vi "write into binary.vi"() -> ()   [LabVIEW 2012]
uses:
  <vilib>/rvi/interface/nirviOpenFPGA/nirviOpenFPGA.xnode
  <vilib>/rvi/interface/nirviMethod/nirviMethod.xnode
  <vilib>/rvi/errors/niLvFpgaMergeErrorWithErrorCode.vi
  <vilib>/ptbypt/NI_PtbyPt.lvlib
  <vilib>/rvi/interface/nirviCloseFPGA/nirviCloseFPGA.xnode
  <vilib>/rvi/interface/nirviReadWriteControl/nirviReadWriteControl.xnode
  <vilib>/rvi/interface/Simulation/niFpgaSimulationCallBeginRW.vi
  <vilib>/rvi/errors/niLvFpgaAdjustHostInterfaceError.vi
  <vilib>/FPGAPlugInAG/Dynamic/niLvFpga_Run_Dynamic.vi
  FPGA Bitfiles/Mockup_FPGATarget_TopLevelFPGAtryw_gkKwyDHwWeY.lvbitx
  <vilib>/FPGAPlugInAG/Dynamic/niLvFpga_StartFifo_Dynamic.vi
  <vilib>/LabVIEW Targets/FPGA/FlexRIO/CustomFPGAMethods/79XXR_Method_IOModuleStatusImpl.vi
  <vilib>/FPGAPlugInAG/Dynamic/niLvFpga_Close_Dynamic.vi
  <vilib>/FPGAPlugInAG/PXI-7951R/niLvFpga_Open_PXI-7951R.vi
  <vilib>/rvi/interface/common/dynamic/niFpgaDynamicAddResources.vi
  <vilib>/FPGAPlugInAG/Dynamic/niLvFpga_ConfigureFifo_Dynamic.vi
  <vilib>/FPGAPlugInAG/Dynamic/niLvFpga_ReadFifo_Dynamic.vi
  <vilib>/userdefined/High Color/nirio_resource_hc.ctl
panel:
  in  "det_type":string[](array[string])
  in  "voltage":string[](array[string])
  in  "Serial numbers":string[](array[string])
  in  "Sources":string[](array[string])
  in  "stop 2":bool
  in  "show_trigger_position_for_debugging":bool
  in  "PXI address":T1 caption="RIO Device"
  in  "Channel 8":bool caption="Channel 1"
  in  "Channel 7":bool caption="Channel 1"
  in  "Channel 6":bool caption="Channel 1"
  in  "Channel 5":bool caption="Channel 1"
  in  "Channel 4":bool caption="Channel 1"
  in  "Channel 3":bool caption="Channel 1"
  in  "Channel 2":bool caption="Channel 1"
  in  "Channel 1":bool
  out "XML String":string
  in  "Trigger":i16[](array[numeric])=[4000, 4000, 4000, 4000, 4000, 4000, 4000, 4000]
  in  "number_of_arrays_per_file":u32=1000
  in  "File Path":path=path "D:/Users/mkurz/Desktop/test data from the FPGA/data from the new program of Drew"
  out "error out":errorcluster
  in  "samples_dataonly":u32=95
  in  "with dead time":bool
  in  "circular buffer length":u32=1000
  in  "pretrigger_samples":u32=15
  in  "number_of_samples_per_array":u32=500000 format="%.2p"
  in  "Simulate":bool
  in  "stop":bool
  out "Elements in FIFO":u32(graph)
  out "Data":i16[](graph)
  out "Inst. Throughput":dbl format="%#_6p"
  out "Loop Time":u32
  in  "read_rate_ms":u32=50
  out "Average Throughput":dbl(graph)
  in  "Write to Disk":bool
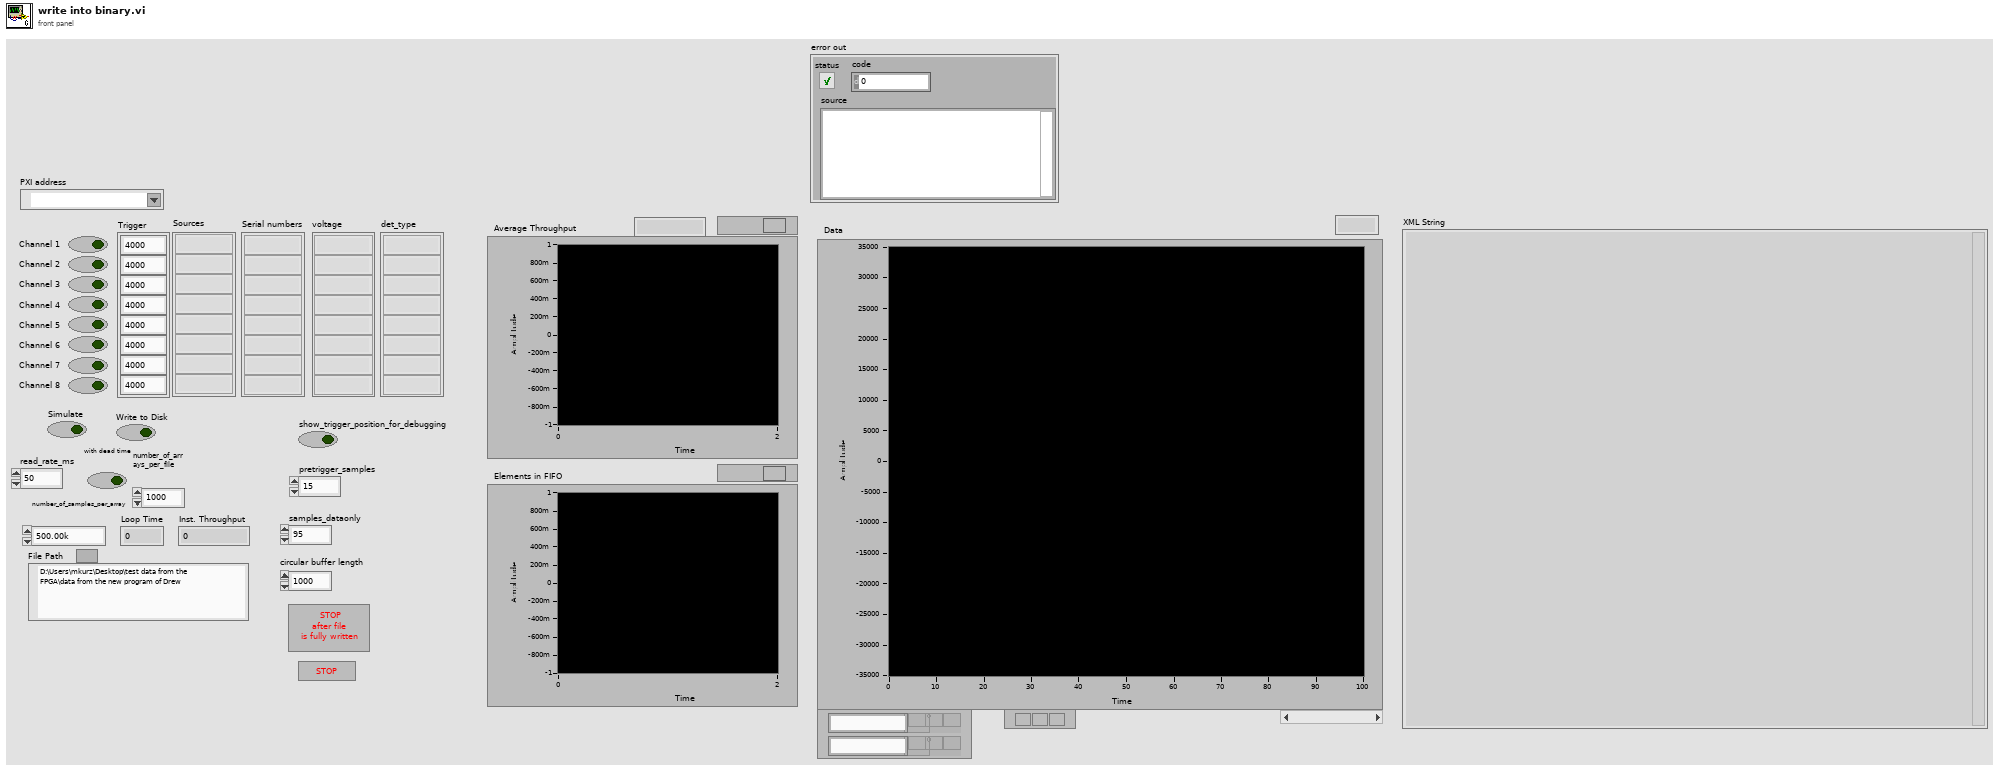
[diagram p1: front panel]
types:
  T1 = typedef "nirio_resource_hc.ctl" = tag
  T2 = enum16{"open", "replace", "create", "open or create", "replace or create", "replace or create with confirmation"}
  T3 = enum16{"big-endian, network order", "native, host order", "little-endian"}
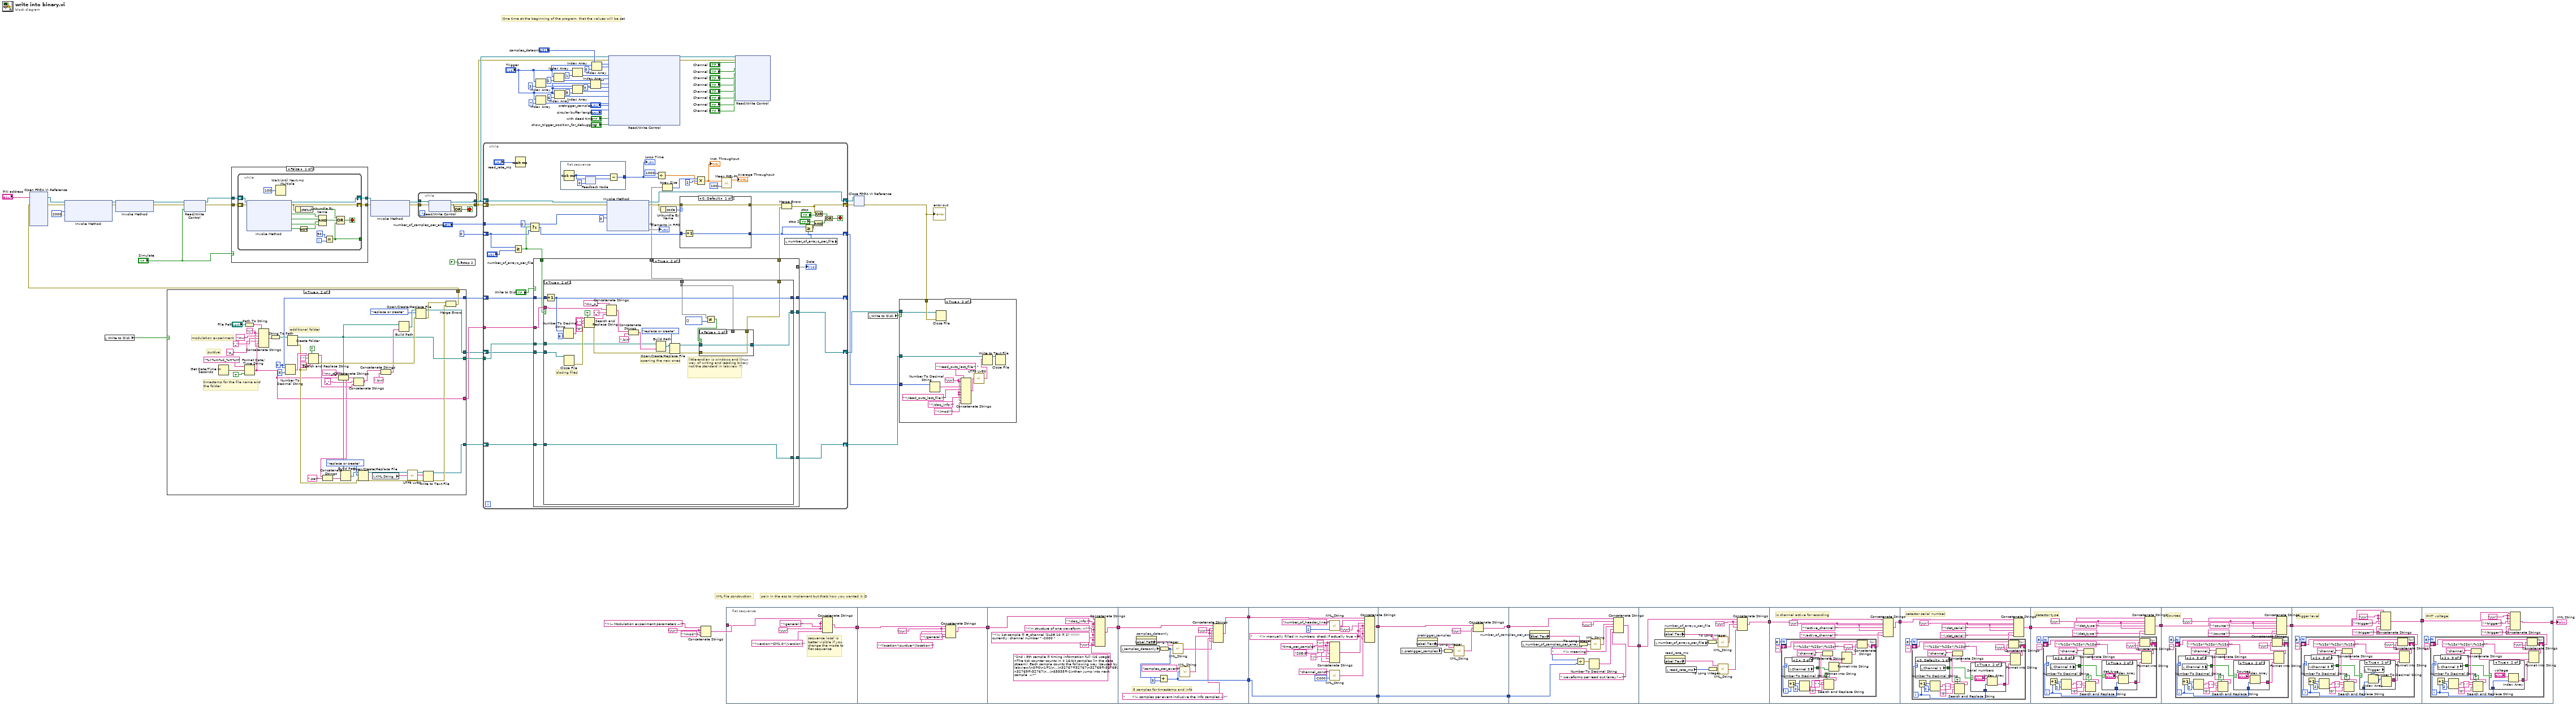
[diagram p0: block diagram]
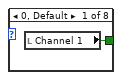
[diagram p2: hidden frame]
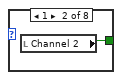
[diagram p3: hidden frame]
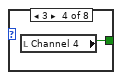
[diagram p4: hidden frame]
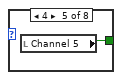
[diagram p5: hidden frame]
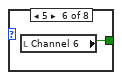
[diagram p6: hidden frame]
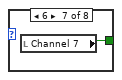
[diagram p7: hidden frame]
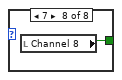
[diagram p8: hidden frame]
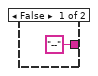
[diagram p9: hidden frame]
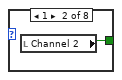
[diagram p10: hidden frame]
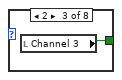
[diagram p11: hidden frame]
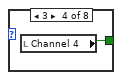
[diagram p12: hidden frame]
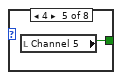
[diagram p13: hidden frame]
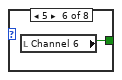
[diagram p14: hidden frame]
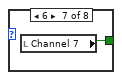
[diagram p15: hidden frame]
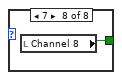
[diagram p16: hidden frame]
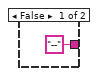
[diagram p17: hidden frame]
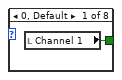
[diagram p18: hidden frame]
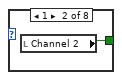
[diagram p19: hidden frame]
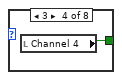
[diagram p20: hidden frame]
diagram:
  w22 = "\r\n"
  # "pain in the ass to implement but thats how you wanted it :D"
  # "XML file construction"
  # "One time at the beginning of the program, that the values will be set"
  n1 = local read "Write to Disk"() -> (w65:bool)
  n2 = case shown="True" w65 {
    tunnel: [_ w107] -> w70
    tunnel: [_ w95] -> w69
    tunnel: [_ w109] -> w68
    tunnel: [_ w115] -> w66
    tunnel: [_ w111] -> w64
    tunnel: [_ w97] -> w62
    frame False {
    }
    frame True {
      w115 = 0 ("number")
      w96 = "\\" ("string")
      # "modulation experiment"
      # "purdue"
      # "timestamp for the file name and the folder"
      # "additional folder"
      n3 = Get Date/Time In Seconds() -> (seconds since 1Jan1904=w124:timestamp)
      n4 = Path To String(path="File Path") -> (string=w126:string)
      n5 = Format Date/Time String(time format string (%c)="%Y%m%d_%H%M", seconds (now)=w124, UTC format=TRUE) -> (date/time string=w95:string)
      n6 = Concatenate Strings(w126, w96, "mx" ("string"), "_" ("string"), "p_" ("string"), w95, w96) -> (w129:string)
      n7 = String To Path(string=w129) -> (path=w130:path)
      n8 = Number To Decimal String(number=w115, width (-)=i16 6) -> (decimal integer string=w119:string)
      n9 = Create Folder(path (use dialog)=w130) -> (created path=w107:path, error out=w105:errorcluster)  [unwired: 2 in, 1 out]
      n10 = Search and Replace String(replace all?=TRUE ("replace all? (F)"), input string=w119, search string=" ", replace string="0" ("replace string (\"\")"), error in=w105) -> (result string=w91:string, error out=w113:errorcluster)  [unwired: 3 in, 2 out]
      n11 = Concatenate Strings("mx_p_" ("string"), w95) -> (w92:string)
      n12 = Concatenate Strings(w92, ".par" ("substring (\"\")")) -> (w102:string)
      n13 = Build Path(base path=w107, name or relative path=w102) -> (appended path=w108:path)
      n14 = Concatenate Strings(w92, "_" ("string"), w91) -> (w93:string)
      n15 = Open/Create/Replace File(file path (use dialog)=w108, error in=w105, operation (0:open)=T2."replace or create") -> (refnum out=w98:refnum<file>, error out=w100:errorcluster)  [unwired: 3 in, 1 out]
      n16 = local read "XML String"() -> (w88:string)
      n17 = Concatenate Strings(w93, ".bin" ("substring (\"\")")) -> (w104:string)
      n18 = Build Path(base path=w107, name or relative path=w104) -> (appended path=w114:path)
      n19 = call "UTF8 LV80.vi"("text"=w88) -> ("utf-8 text out"=w89:string)
      n20 = Open/Create/Replace File(file path (use dialog)=w114, error in=w113, operation (0:open)=T2."replace or create") -> (refnum out=w111:refnum<file>, error out=w110:errorcluster)  [unwired: 3 in, 1 out]
      n21 = Write to Text File(file (use dialog)=w98, text=w89, error in=w100) -> (refnum out=w97:refnum<file>, error out=w99:errorcluster)  [unwired: 1 in, 1 out]
      n22 = Merge Errors(w110, w99) -> (w109:errorcluster)
    }
  }
  n23 = xnode "Open FPGA VI Reference"("error in"=w68, "resource name"="PXI address") -> ("FPGA VI Reference Out"=w83:refnum<k20>, "error out"=w82:errorcluster)
  n24 = xnode "Invoke Method"("FPGA VI Reference In"=w83, "error in"=w82, "Requested Depth"=u32 20000000) -> ("FPGA VI Reference Out"=w85:refnum<k20>, "error out"=w84:errorcluster)  [unwired: 1 out]
  n25 = xnode "Invoke Method"("FPGA VI Reference In"=w85, "error in"=w84) -> ("FPGA VI Reference Out"=w77:refnum<k20>, "error out"=w76:errorcluster)
  n26 = xnode "Read/Write Control"("FPGA VI Reference In"=w77, "error in"=w76, "Simulate"="Simulate") -> ("FPGA VI Reference Out"=w42:refnum<k20>, "error out"=w41:errorcluster)
  n27 = case shown="False" "Simulate" {
    tunnel: [w134 w152] -> w78
    tunnel: [w133 w151] -> w79
    tunnel: w42 -> [w132 w152]
    tunnel: w41 -> [w131 w151]
    frame False {
      n28 = while {
        shift-right: [w141] -> w133
        shift-left: w131 -> [w149]
        shift-right: [w148] -> w134
        shift-left: w132 -> [w150]
        tunnel: [w137] -> _
        i -> [w143]
        stop <- w138 stop-if-true
        n29 = xnode "Invoke Method"("FPGA VI Reference In"=w150, "error in"=w149) -> ("FPGA VI Reference Out"=w148:refnum<k20>, "error out"=w141:errorcluster, "IO Module Present?"=w147:bool, "Power Enabled?"=w146:bool, "IO Enabled?"=w145:bool, "IO Module Mismatch?"=w136:bool)
        n30 = Wait Until Next ms Multiple(millisecond multiple=u32 100) -> ()  [unwired: 1 out]
        n31 = Unbundle By Name(w141) -> ("status"=w140:bool)
        n32 = Not(x=w136) -> (.not. x?=w135:bool)
        n33 = Compound Arithmetic op=AND(w147, w146, w145, w135) -> (w139:bool)
        n34 = Equal?(x=50, y=w143) -> (x = y?=w137:bool)
        n35 = Compound Arithmetic op=OR(w140, w139, w137) -> (w138:bool)
      }
    }
    frame True {
    }
  }
  n36 = xnode "Invoke Method"("FPGA VI Reference In"=w78, "error in"=w79) -> ("FPGA VI Reference Out"=w80:refnum<k20>, "error out"=w81:errorcluster)  [unwired: 1 in]
  n37 = while {
    tunnel: [w153] -> w25
    tunnel: [w158] -> w26
    tunnel: w80 -> [w157]
    tunnel: w81 -> [w156]
    stop <- w154 stop-if-true
    n38 = xnode "Read/Write Control"("FPGA VI Reference In"=w157, "error in"=w156) -> ("FPGA VI Reference Out"=w158:refnum<k20>, "error out"=w153:errorcluster, "Init Done"=w155)
    n39 = Or(x=w153, y=w155) -> (x .or. y?=w154:bool)
  }
  n40 = local write "stop 2"(FALSE ("stop 2")) -> ()
  n41 = while {
    shift-right: [w202] -> w87
    shift-left: w26 -> [w186]
    shift-right: [w175] -> w86
    shift-left: w25 -> [w185]
    tunnel: "number_of_samples_per_array" -> [w187]
    tunnel: w69 -> [w183]
    shift-right: [w162] -> w27
    shift-left: u32 0 -> [w182]
    tunnel: w70 -> [w184]
    shift-right: [w177] -> _
    shift-left: w66 -> [w178]
    shift-right: [w172] -> w63
    shift-left: w64 -> [w173]
    shift-right: [w169] -> w61
    shift-left: w62 -> [w170]
    stop <- w159 stop-if-true
    n42 = Greater Or Equal?(x=w182, y="number_of_arrays_per_file") -> (x >= y?=w179:bool)
    n43 = Wait (ms)(milliseconds to wait="read_rate_ms") -> ()  [unwired: 1 out]
    n44 = Select(t=u32 0, s=w179, f=w182) -> (s? t:f=w180:u32)
    n45 = flat-sequence {
      tunnel: [w206] -> w191
      frame #0 {
        n46 = Tick Count (ms)() -> (millisecond timer value=w205:u32)
        n47 = feedback #1(u32 0 ("millisecond timer value")) -> (w204:u32)
        n48 = feedback-in #1(w205) -> ()
        n49 = Subtract(x=w205, y=w204) -> (x-y=w206:u32)
      }
    }
    n50 = xnode "Invoke Method"("FPGA VI Reference In"=w186, "error in"=w185, "Number of Elements"=w187, "Timeout (ms)"=0) -> ("FPGA VI Reference Out"=w202:refnum<k20>, "error out"=w198:errorcluster, "Data"=w166:void[], "Elements Remaining"=→"Elements in FIFO")
    n51 = case shown="True" "Write to Disk" {
      tunnel: w166 -> [w208 w213]
      tunnel: [w208 _] -> w167
      tunnel: w184 -> [_ w221]
      tunnel: w183 -> [_ w220]
      tunnel: w179 -> [_ w219]
      tunnel: w178 -> [w210 w218]
      tunnel: [w210 w217] -> w177
      tunnel: [_ w216] -> w174
      tunnel: [w209 w215] -> w172
      tunnel: w173 -> [w209 w214]
      tunnel: w170 -> [w207 w212]
      tunnel: [w207 w211] -> w169
      frame False {
      }
      frame True {
        n52 = case shown="True" w219 {
          tunnel: w221 -> [_ w241]
          tunnel: w220 -> [_ w246]
          tunnel: w213 -> [w224 w238]
          tunnel: [w222 w236] -> w216
          tunnel: w214 -> [w228 w254]
          tunnel: w218 -> [w229 w256]
          tunnel: [w229 w255] -> w217
          tunnel: [w227 w247] -> w215
          tunnel: w212 -> [w226 w237]
          tunnel: [w226 w237] -> w211
          frame False {
            # "binary writing will write 0 if there is no data"
            n53 = Not Equal?(x=w224, y=i16[] []) -> (x != y?=w223:bool)
            n54 = case shown="False" w223 {
              tunnel: w228 -> [w230 w235]
              tunnel: [w230 w234] -> w227
              tunnel: [_ w233] -> w222
              tunnel: w224 -> [_ w231]
              frame False {
              }
              frame True {
                n55 = Write to Binary File(file (use dialog)=w235, data=w231, 9:T3."little-endian" ("byte order (0:big-endian, network order)")) -> (refnum out=w234:refnum<file>, error out=w233:errorcluster)  [unwired: 3 in, 1 out]
              }
            }
          }
          frame True {
            # "opening the new ones"
            # "closing files"
            # "little-endian is windows and linux way of writing and reading binary not the standard in labview !?!"
            n56 = Increment(x=w256) -> (x+1=w255:i32)
            n57 = Number To Decimal String(number=w255, width (-)=i16 6) -> (decimal integer string=w258:string)
            n58 = Close File(refnum=w254) -> (error out=w253:errorcluster)  [unwired: 1 in, 1 out]
            n59 = Search and Replace String(replace all?=TRUE ("replace all? (F)"), input string=w258, search string=" ", replace string="0" ("replace string (\"\")"), error in=w253) -> (result string=w245:string, error out=w252:errorcluster)  [unwired: 3 in, 2 out]
            n60 = Concatenate Strings("mx_p_" ("string"), w246, "_" ("string"), w245) -> (w242:string)
            n61 = Concatenate Strings(w242, ".bin" ("substring (\"\")")) -> (w243:string)
            n62 = Build Path(base path=w241, name or relative path=w243) -> (appended path=w251:path)
            n63 = Open/Create/Replace File(file path (use dialog)=w251, error in=w252, operation (0:open)=T2."replace or create") -> (refnum out=w248:refnum<file>, error out=w249:errorcluster)  [unwired: 3 in, 1 out]
            n64 = Not Equal?(x=w238, y=i16[] []) -> (x != y?=w239:bool)
            n65 = case shown="False" w239 {
              tunnel: w249 -> [w264 w271]
              tunnel: w248 -> [w265 w270]
              tunnel: [w265 w269] -> w247
              tunnel: [w264 w268] -> w236
              tunnel: w238 -> [_ w267]
              frame False {
              }
              frame True {
                n66 = Write to Binary File(file (use dialog)=w270, data=w267, error in=w271, 9:T3."little-endian" ("byte order (0:big-endian, network order)")) -> (refnum out=w269:refnum<file>, error out=w268:errorcluster)  [unwired: 2 in, 1 out]
              }
            }
          }
        }
      }
    }
    "Data" <- w167
    n67 = Divide(x=u32 1000, y=w191) -> (x/y=w193:dbl)
    n68 = Unbundle By Name(w198) -> ("code"=w199:i32)
    n69 = Array Size(array=w166) -> (size(s)=w197:i32)
    n70 = case shown="0, Default" w199 {
      tunnel: [w274 errorcluster {"status"=FALSE, "code"=0, "source"=""} ("error constant")] -> w176
      tunnel: w198 -> [w274 _]
      tunnel: w180 -> [w273 w275]
      tunnel: [w272 w275] -> w162
      frame 0, Default {
        n71 = Increment(x=w273) -> (x+1=w272:u32)
      }
      frame -50400 {
      }
    }
    n72 = Compound Arithmetic op=MULTIPLY(w197, 2 ("y"), w193) -> (w189:dbl)
    "Inst. Throughput" <- w189
    n73 = call <vilib>:"Mean PtByPt.vi"("x"=w189, "sample length"=100) -> ("mean"=→"Average Throughput":dbl)  [unwired: 2 in, 1 out]
    n74 = Merge Errors(w176, w174) -> (w175:errorcluster)
    n75 = local read "number_of_arrays_per_file"() -> (w165:u32)
    n76 = Greater Or Equal?(x=w162, y=w165) -> (x >= y?=w164:bool)
    n77 = And(x="stop 2", y=w164) -> (x .and. y?=w163:bool)
    n78 = Or(x=w175, y="stop") -> (x .or. y?=w160:bool)
    n79 = Or(x=w160, y=w163) -> (x .or. y?=w159:bool)
    "Loop Time" <- w191
  }
  n80 = Index Array(array="Trigger", index=3) -> (element=w51:i16)
  n81 = Index Array(array="Trigger", index=7) -> (element=w43:i16)
  n82 = Index Array(array="Trigger", index=2) -> (element=w54:i16)
  n83 = Index Array(array="Trigger", index=6) -> (element=w44:i16)
  n84 = Index Array(array="Trigger", index=1) -> (element=w53:i16)
  n85 = Index Array(array="Trigger", index=5) -> (element=w45:i16)
  n86 = Index Array(array="Trigger", index=4) -> (element=w46:i16)
  n87 = Index Array(array="Trigger", index=0) -> (element=w38:i16)
  n88 = xnode "Read/Write Control"("FPGA VI Reference In"=w26, "error in"=w25, "Record Size only data"="samples_dataonly", "Trigger 1"=w38, "Trigger 2"=w53, "Trigger 3"=w54, "Trigger 4"=w51, "Trigger 5"=w46, "Trigger 6"=w45, "Trigger 7"=w44, "Trigger 8"=w43, "# of pretrigger"="pretrigger_samples", "circular buffer length"="circular buffer length", "with dead time"="with dead time", "show_trigger_position_for_debugging"="show_trigger_position_for_debugging") -> ("FPGA VI Reference Out"=w40:refnum<k20>, "error out"=w39:errorcluster)
  n89 = Concatenate Strings("<!-- Modulation experiment parameters -->", w22, w22, "<mod>" ("string")) -> (w23:string)
  n90 = flat-sequence {
    tunnel: w23 -> [w278]
    tunnel: [w280] -> w17
    tunnel: w17 -> [w284]
    tunnel: [w286] -> w16
    tunnel: w16 -> [w287]
    tunnel: [w293] -> w15
    tunnel: w15 -> [w301]
    tunnel: [w302] -> w4
    tunnel: [w297] -> w2
    tunnel: w4 -> [w320]
    tunnel: [w321] -> w3
    tunnel: w2 -> [w322]
    tunnel: [w322] -> w1
    tunnel: w3 -> [w328]
    tunnel: [w327] -> w14
    tunnel: [w323] -> w5
    tunnel: w1 -> [w323]
    tunnel: w14 -> [w338]
    tunnel: [w337] -> w13
    tunnel: w5 -> [w331]
    tunnel: w13 -> [w349]
    tunnel: [w351] -> w12
    tunnel: w12 -> [w361]
    tunnel: [w354] -> w11
    tunnel: w11 -> [w394]
    tunnel: [w387] -> w9
    tunnel: w9 -> [w425]
    tunnel: [w424] -> w8
    tunnel: w8 -> [w462]
    tunnel: [w461] -> w7
    tunnel: [w505] -> w10
    tunnel: w7 -> [w498]
    tunnel: w10 -> [w537]
    tunnel: [w536] -> w6
    frame #0 {
      w277 = "\r\n"
      # "sequence local is better visible if you change the mode to flat sequence"
      n91 = Concatenate Strings(w278, w277, w277, "<general>" ("string"), w277, "<version>CM1.0</version>" ("string")) -> (w280:string)
    }
    frame #1 {
      w283 = "\r\n"
      n92 = Concatenate Strings(w284, w283, "<location>purdue</location>" ("string"), w283, "</general>" ("string")) -> (w286:string)
    }
    frame #2 {
      w288 = "\r\n"
      n93 = Concatenate Strings(w287, w288, w288, "<daq_info>" ("string"), w288, "<!-- structure of one waveform: -->", w288, "<!-- 1st sample = #_channel (2LSB 10 = 2) !!!!!!!! currently: channel number * -2000 " ("string"), w288, "2nd - 5th sample = timing information full I16 usage\nThe tick counter counts in 4 16-bit samples (in the data stream). Each sample counts the following way (caused by labview)\n0=0\n1=1\n…\n32767=32767\n32768=-32768\n32769=-32767\n…\n65535=-1\nthen jump into next sample  -->" ("string"), w288) -> (w293:string)
    }
    frame #3 {
      w294 = "\r\n"
      # "5 samples for timestamp and info"
      n94 = local read "samples_dataonly"() -> (w305:u32)
      n95 = property on="samples_dataonly" class="DigNum (strict)"() -> ("Label.Text"=w304:string)  [unwired: 2 in, 2 out]
      n96 = To Long Integer(number=w305) -> (32bit integer=w299:i32)
      n97 = Add(x=w299, y=5) -> (x+y=w297:i32)
      n98 = call "XML_String.vi"("variable"=w299, "variable name"=w304) -> ("xml string"=w303:string)  [unwired: 1 in]
      n99 = call "XML_String.vi"("variable"=w297, "variable name"="samples_per_event") -> ("xml string"=w296:string)  [unwired: 1 in]
      n100 = Concatenate Strings(w301, w294, w303, w294, w296, "      <!-- samples per event inclusive the info samples -->" ("string"), w294) -> (w302:string)
    }
    frame #4 {
      w313 = ">" ("string")
      w316 = "<" ("string")
      w314 = "time_per_sample" ("variable name")
      w307 = "      <!-- manually filled in numbers, check if actually true -->" ("string")
      w306 = "\r\n"
      n101 = call "XML_String.vi"("variable"=-2000, "variable name"="channel_const") -> ("xml string"=w308:string)  [unwired: 1 in]
      n102 = call "XML_String.vi"("variable"=2, "variable name"="number_of_header_lines") -> ("xml string"=w319:string)  [unwired: 1 in]
      n103 = Concatenate Strings(w316, w314, w313, "20E-9" ("string"), w316, "/" ("string"), w314, w313) -> (w311:string)
      n104 = Concatenate Strings(w320, w319, w307, w306, w311, w307, w306, w308, w307, w306) -> (w321:string)
    }
    frame #5 {
      n105 = local read "pretrigger_samples"() -> (w330:u32)
      n106 = property on="pretrigger_samples" class="DigNum (strict)"() -> ("Label.Text"=w329:string)  [unwired: 2 in, 2 out]
      n107 = To Long Integer(number=w330) -> (32bit integer=w326:i32)
      n108 = call "XML_String.vi"("variable"=w326, "variable name"=w329) -> ("xml string"=w324:string)  [unwired: 1 in]
      n109 = Concatenate Strings(w328, w324, "\r\n") -> (w327:string)
    }
    frame #6 {
      n110 = local read "number_of_samples_per_array"() -> (w335:u32)
      n111 = property on="number_of_samples_per_array" class="DigNum (strict)"() -> ("Label.Text"=w342:string)  [unwired: 2 in, 2 out]
      n112 = Divide(x=w335, y=w331) -> (x/y=w336:dbl)
      n113 = To Long Integer(number=w335) -> (32bit integer=w339:i32)
      n114 = Number To Decimal String(number=w336) -> (decimal integer string=w333:string)  [unwired: 1 in]
      n115 = call "XML_String.vi"("variable"=w339, "variable name"=w342) -> ("xml string"=w341:string)  [unwired: 1 in]
      n116 = Concatenate Strings(w338, "\r\n", w341, "        <!-- meaning " ("string"), w333, " waveforms per read out (array) -->" ("string")) -> (w337:string)
    }
    frame #7 {
      w347 = "\r\n"
      n117 = local read "number_of_arrays_per_file"() -> (w348:u32)
      n118 = property on="number_of_arrays_per_file" class="DigNum (strict)"() -> ("Label.Text"=w353:string)  [unwired: 2 in, 2 out]
      n119 = property on="read_rate_ms" class="DigNum (strict)"() -> ("Label.Text"=w346:string)  [unwired: 2 in, 2 out]
      n120 = local read "read_rate_ms"() -> (w345:u32)
      n121 = To Long Integer(number=w348) -> (32bit integer=w350:i32)
      n122 = To Long Integer(number=w345) -> (32bit integer=w344:i32)
      n123 = call "XML_String.vi"("variable"=w350, "variable name"=w353) -> ("xml string"=w352:string)  [unwired: 1 in]
      n124 = call "XML_String.vi"("variable"=w344, "variable name"=w346) -> ("xml string"=w343:string)  [unwired: 1 in]
      n125 = Concatenate Strings(w349, w347, w352, w347, w343) -> (w351:string)
    }
    frame #8 {
      w358 = "\r\n"
      # "is channel active for recording"
      n126 = for {
        N: 8 -> [_]
        shift-right: [w367] -> w355
        shift-left: "" -> [w368]
        i -> [w366]
        n127 = case shown="2" w366 {
          tunnel: [w379 w380 w381 w382 w383 w384 w385 w386] -> w363
          frame 0, Default {
            n128 = local read "Channel 1"() -> (w379:bool)
          }
          frame 1 {
            n129 = local read "Channel 2"() -> (w380:bool)
          }
          frame 2 {
            n130 = local read "Channel 3"() -> (w381:bool)
          }
          frame 3 {
            n131 = local read "Channel 4"() -> (w382:bool)
          }
          frame 4 {
            n132 = local read "Channel 5"() -> (w383:bool)
          }
          frame 5 {
            n133 = local read "Channel 6"() -> (w384:bool)
          }
          frame 6 {
            n134 = local read "Channel 7"() -> (w385:bool)
          }
          frame 7 {
            n135 = local read "Channel 8"() -> (w386:bool)
          }
        }
        n136 = Increment(x=w366) -> (x+1=w372:i32)
        n137 = Number To Decimal String(number=w372, width (-)=i16 2) -> (decimal integer string=w375:string)
        n138 = Search and Replace String(replace all?=TRUE ("replace all? (F)"), input string=w375, search string=" ", replace string="0" ("replace string (\"\")")) -> (result string=w370:string)  [unwired: 4 in, 3 out]
        n139 = Concatenate Strings("channel_" ("initial string"), w370) -> (w369:string)
        n140 = Format Into String(w363) -> (resulting string=w362:string)  [unwired: 3 in, 1 out]
        n141 = Format Into String(format string="<%1$s>%2$s</%1$s>", w369, w362) -> (resulting string=w365:string)  [unwired: 2 in, 1 out]
        n142 = Concatenate Strings(w368, w365, "\r\n") -> (w367:string)
      }
      n143 = Concatenate Strings(w361, w358, w358, "<active_channel>" ("string"), w358, w355, "</active_channel>" ("string")) -> (w354:string)
    }
    frame #9 {
      w391 = "\r\n"
      # "setector serial number"
      n144 = for {
        N: 8 -> [_]
        shift-right: [w400] -> w388
        shift-left: "" -> [w401]
        i -> [w396]
        n145 = case shown="0, Default" w396 {
          tunnel: [w416 w417 w418 w419 w420 w421 w422 w423] -> w397
          frame 0, Default {
            n146 = local read "Channel 1"() -> (w416:bool)
          }
          frame 1 {
            n147 = local read "Channel 2"() -> (w417:bool)
          }
          frame 2 {
            n148 = local read "Channel 3"() -> (w418:bool)
          }
          frame 3 {
            n149 = local read "Channel 4"() -> (w419:bool)
          }
          frame 4 {
            n150 = local read "Channel 5"() -> (w420:bool)
          }
          frame 5 {
            n151 = local read "Channel 6"() -> (w421:bool)
          }
          frame 6 {
            n152 = local read "Channel 7"() -> (w422:bool)
          }
          frame 7 {
            n153 = local read "Channel 8"() -> (w423:bool)
          }
        }
        n154 = Increment(x=w396) -> (x+1=w405:i32)
        n155 = Number To Decimal String(number=w405, width (-)=i16 2) -> (decimal integer string=w408:string)
        n156 = Search and Replace String(replace all?=TRUE ("replace all? (F)"), input string=w408, search string=" ", replace string="0" ("replace string (\"\")")) -> (result string=w403:string)  [unwired: 4 in, 3 out]
        n157 = Concatenate Strings("channel_" ("initial string"), w403) -> (w402:string)
        n158 = case shown="True" w397 {
          tunnel: w396 -> [_ w415]
          tunnel: ["--" ("String") w414] -> w395
          frame False {
          }
          frame True {
            n159 = Index Array(array="Serial numbers", index=w415) -> (element=w414:string)
          }
        }
        n160 = Format Into String(format string="<%1$s>%2$s</%1$s>", w402, w395) -> (resulting string=w399:string)  [unwired: 2 in, 1 out]
        n161 = Concatenate Strings(w401, w399, "\r\n") -> (w400:string)
      }
      n162 = Concatenate Strings(w394, w391, w391, "<det_serial>" ("string"), w391, w388, "</det_serial>" ("string")) -> (w387:string)
    }
    frame #10 {
      w428 = "\r\n"
      # "detector type"
      n163 = for {
        N: 8 -> [_]
        shift-right: [w437] -> w431
        shift-left: "" -> [w438]
        i -> [w433]
        n164 = case shown="2" w433 {
          tunnel: [w453 w454 w455 w456 w457 w458 w459 w460] -> w434
          frame 0, Default {
            n165 = local read "Channel 1"() -> (w453:bool)
          }
          frame 1 {
            n166 = local read "Channel 2"() -> (w454:bool)
          }
          frame 2 {
            n167 = local read "Channel 3"() -> (w455:bool)
          }
          frame 3 {
            n168 = local read "Channel 4"() -> (w456:bool)
          }
          frame 4 {
            n169 = local read "Channel 5"() -> (w457:bool)
          }
          frame 5 {
            n170 = local read "Channel 6"() -> (w458:bool)
          }
          frame 6 {
            n171 = local read "Channel 7"() -> (w459:bool)
          }
          frame 7 {
            n172 = local read "Channel 8"() -> (w460:bool)
          }
        }
        n173 = Increment(x=w433) -> (x+1=w442:i32)
        n174 = Number To Decimal String(number=w442, width (-)=i16 2) -> (decimal integer string=w445:string)
        n175 = Search and Replace String(replace all?=TRUE ("replace all? (F)"), input string=w445, search string=" ", replace string="0" ("replace string (\"\")")) -> (result string=w440:string)  [unwired: 4 in, 3 out]
        n176 = Concatenate Strings("channel_" ("initial string"), w440) -> (w439:string)
        n177 = case shown="True" w434 {
          tunnel: w433 -> [_ w452]
          tunnel: ["--" ("String") w451] -> w432
          frame False {
          }
          frame True {
            n178 = Index Array(array="det_type", index=w452) -> (element=w451:string)
          }
        }
        n179 = Format Into String(format string="<%1$s>%2$s</%1$s>", w439, w432) -> (resulting string=w436:string)  [unwired: 2 in, 1 out]
        n180 = Concatenate Strings(w438, w436, "\r\n") -> (w437:string)
      }
      n181 = Concatenate Strings(w425, w428, w428, "<det_type>" ("string"), w428, w431, "</det_type>" ("string")) -> (w424:string)
    }
    frame #11 {
      w465 = "\r\n"
      # "Sources"
      n182 = for {
        N: 8 -> [_]
        shift-right: [w474] -> w468
        shift-left: "" -> [w475]
        i -> [w470]
        n183 = case shown="2" w470 {
          tunnel: [w490 w491 w492 w493 w494 w495 w496 w497] -> w471
          frame 0, Default {
            n184 = local read "Channel 1"() -> (w490:bool)
          }
          frame 1 {
            n185 = local read "Channel 2"() -> (w491:bool)
          }
          frame 2 {
            n186 = local read "Channel 3"() -> (w492:bool)
          }
          frame 3 {
            n187 = local read "Channel 4"() -> (w493:bool)
          }
          frame 4 {
            n188 = local read "Channel 5"() -> (w494:bool)
          }
          frame 5 {
            n189 = local read "Channel 6"() -> (w495:bool)
          }
          frame 6 {
            n190 = local read "Channel 7"() -> (w496:bool)
          }
          frame 7 {
            n191 = local read "Channel 8"() -> (w497:bool)
          }
        }
        n192 = Increment(x=w470) -> (x+1=w479:i32)
        n193 = Number To Decimal String(number=w479, width (-)=i16 2) -> (decimal integer string=w482:string)
        n194 = Search and Replace String(replace all?=TRUE ("replace all? (F)"), input string=w482, search string=" ", replace string="0" ("replace string (\"\")")) -> (result string=w477:string)  [unwired: 4 in, 3 out]
        n195 = Concatenate Strings("channel_" ("initial string"), w477) -> (w476:string)
        n196 = case shown="True" w471 {
          tunnel: w470 -> [_ w489]
          tunnel: ["--" ("String") w488] -> w469
          frame False {
          }
          frame True {
            n197 = Index Array(array="Sources", index=w489) -> (element=w488:string)
          }
        }
        n198 = Format Into String(format string="<%1$s>%2$s</%1$s>", w476, w469) -> (resulting string=w473:string)  [unwired: 2 in, 1 out]
        n199 = Concatenate Strings(w475, w473, "\r\n") -> (w474:string)
      }
      n200 = Concatenate Strings(w462, w465, w465, "<source>" ("string"), w465, w468, "</source>" ("string")) -> (w461:string)
    }
    frame #12 {
      w503 = "\r\n"
      # "Trigger level"
      n201 = for {
        N: 8 -> [_]
        shift-right: [w511] -> w499
        shift-left: "" -> [w512]
        i -> [w507]
        n202 = case shown="2" w507 {
          tunnel: [w528 w529 w530 w531 w532 w533 w534 w535] -> w508
          frame 0, Default {
            n203 = local read "Channel 1"() -> (w528:bool)
          }
          frame 1 {
            n204 = local read "Channel 2"() -> (w529:bool)
          }
          frame 2 {
            n205 = local read "Channel 3"() -> (w530:bool)
          }
          frame 3 {
            n206 = local read "Channel 4"() -> (w531:bool)
          }
          frame 4 {
            n207 = local read "Channel 5"() -> (w532:bool)
          }
          frame 5 {
            n208 = local read "Channel 6"() -> (w533:bool)
          }
          frame 6 {
            n209 = local read "Channel 7"() -> (w534:bool)
          }
          frame 7 {
            n210 = local read "Channel 8"() -> (w535:bool)
          }
        }
        n211 = Increment(x=w507) -> (x+1=w516:i32)
        n212 = Number To Decimal String(number=w516, width (-)=i16 2) -> (decimal integer string=w519:string)
        n213 = Search and Replace String(replace all?=TRUE ("replace all? (F)"), input string=w519, search string=" ", replace string="0" ("replace string (\"\")")) -> (result string=w514:string)  [unwired: 4 in, 3 out]
        n214 = Concatenate Strings("channel_" ("initial string"), w514) -> (w513:string)
        n215 = case shown="True" w508 {
          tunnel: w507 -> [_ w527]
          tunnel: ["--" ("String") w524] -> w506
          frame False {
          }
          frame True {
            n216 = local read "Trigger"() -> (w526:i16[])
            n217 = Index Array(array=w526, index=w527) -> (element=w525:i16)
            n218 = Number To Decimal String(number=w525) -> (decimal integer string=w524:string)  [unwired: 1 in]
          }
        }
        n219 = Format Into String(format string="<%1$s>%2$s</%1$s>", w513, w506) -> (resulting string=w510:string)  [unwired: 2 in, 1 out]
        n220 = Concatenate Strings(w512, w510, "\r\n") -> (w511:string)
      }
      n221 = Concatenate Strings(w498, w503, w503, "<trigger>" ("string"), w503, w499, "</trigger>" ("string")) -> (w505:string)
    }
    frame #13 {
      w539 = "\r\n"
      # "PMT voltage"
      n222 = for {
        N: 8 -> [_]
        shift-right: [w549] -> w543
        shift-left: "" -> [w550]
        i -> [w545]
        n223 = case shown="2" w545 {
          tunnel: [w565 w566 w567 w568 w569 w570 w571 w572] -> w546
          frame 0, Default {
            n224 = local read "Channel 1"() -> (w565:bool)
          }
          frame 1 {
            n225 = local read "Channel 2"() -> (w566:bool)
          }
          frame 2 {
            n226 = local read "Channel 3"() -> (w567:bool)
          }
          frame 3 {
            n227 = local read "Channel 4"() -> (w568:bool)
          }
          frame 4 {
            n228 = local read "Channel 5"() -> (w569:bool)
          }
          frame 5 {
            n229 = local read "Channel 6"() -> (w570:bool)
          }
          frame 6 {
            n230 = local read "Channel 7"() -> (w571:bool)
          }
          frame 7 {
            n231 = local read "Channel 8"() -> (w572:bool)
          }
        }
        n232 = Increment(x=w545) -> (x+1=w554:i32)
        n233 = Number To Decimal String(number=w554, width (-)=i16 2) -> (decimal integer string=w557:string)
        n234 = Search and Replace String(replace all?=TRUE ("replace all? (F)"), input string=w557, search string=" ", replace string="0" ("replace string (\"\")")) -> (result string=w552:string)  [unwired: 4 in, 3 out]
        n235 = Concatenate Strings("channel_" ("initial string"), w552) -> (w551:string)
        n236 = case shown="True" w546 {
          tunnel: w545 -> [_ w564]
          tunnel: ["--" ("String") w563] -> w544
          frame False {
          }
          frame True {
            n237 = Index Array(array="voltage", index=w564) -> (element=w563:string)
          }
        }
        n238 = Format Into String(format string="<%1$s>%2$s</%1$s>", w551, w544) -> (resulting string=w548:string)  [unwired: 2 in, 1 out]
        n239 = Concatenate Strings(w550, w548, "\r\n") -> (w549:string)
      }
      n240 = Concatenate Strings(w537, w539, w539, "<trigger>" ("string"), w539, w543, "</trigger>" ("string")) -> (w536:string)
    }
  }
  n241 = xnode "Read/Write Control"("FPGA VI Reference In"=w40, "error in"=w39, "channel on/off"="Channel 1", "channel 2 on/off"="Channel 2", "channel 3 on/off"="Channel 3", "channel 4 on/off"="Channel 4", "channel 5 on/off"="Channel 5", "channel 6 on/off"="Channel 6", "channel 7 on/off"="Channel 7", "channel 8 on/off"="Channel 8") -> ()  [unwired: 2 out]
  n242 = xnode "Close FPGA VI Reference"("FPGA VI Reference In"=w87, "error in"=w86) -> ("error out"=w73:errorcluster)
  "error out" <- w73
  n243 = local read "Write to Disk"() -> (w71:bool)
  n244 = case shown="True" w71 {
    tunnel: w73 -> [_ w585]
    tunnel: w63 -> [_ w584]
    tunnel: w61 -> [_ w583]
    tunnel: w27 -> [_ w578]
    frame False {
    }
    frame True {
      w576 = "\r\n"
      n245 = Number To Decimal String(number=w578) -> (decimal integer string=w580:string)  [unwired: 1 in]
      n246 = Close File(refnum=w584, error in=w585) -> ()  [unwired: 2 out]
      n247 = Concatenate Strings(w576, w576, "<read_outs_last_file> " ("text"), w580, "</read_outs_last_file>" ("string"), w576, w576, "</daq_info>" ("string"), w576, "</mod>" ("string")) -> (w574:string)
      n248 = call "UTF8 LV80.vi"("text"=w574) -> ("utf-8 text out"=w573:string)
      n249 = Write to Text File(file (use dialog)=w583, text=w573) -> (refnum out=w582:refnum<file>)  [unwired: 2 in, 2 out]
      n250 = Close File(refnum=w582) -> ()  [unwired: 1 in, 2 out]
    }
  }
  "XML String" <- w6
